vi "例8.1 单点模入采集直流电压.vi"() -> ()   [LabVIEW 2017]
panel:
  out "仪表":dbl(knob) scale=0.0..5.0
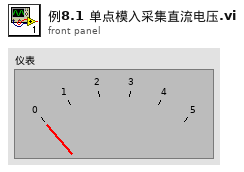
[diagram p1: front panel]
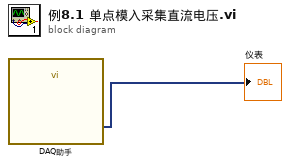
[diagram p0: block diagram]
diagram:
  n1 = call "DAQ助手"() -> ("data"=→"仪表":dynamicdata)  [unwired: 17 in, 2 out]
